vi "Calc Index.vi"(9 "Cols Per Row":i32, 10 "Col":i32, 11 "Row":i32) -> (3 "Index":i32)   [LabVIEW 2020, in "3D (FPGA).lvlib"]
uses:
  3D (FPGA).lvlib
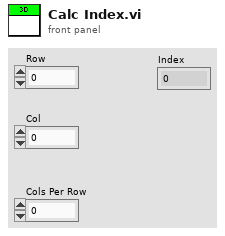
[diagram p1: front panel]
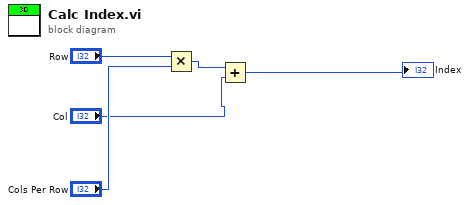
[diagram p0: block diagram]
diagram:
  n1 = Multiply(x="Row", y="Cols Per Row") -> (x*y=w3:i32)
  n2 = Add(x=w3, y="Col") -> (x+y=→"Index":i32)
